vi "Read Message.vi"(4 "timeout in ms (100)":i32=100, 8 "error in (no error)":errorcluster, 11 "RemoteControl.STM in":refnum<class "RemoteControl.STM.lvclass">) -> (0 "error out":errorcluster, 1 "Message ID":u32, 2 "Message":T1, 3 "RemoteControl.STM out":refnum<class "RemoteControl.STM.lvclass">)   [LabVIEW 2016, in "RemoteControl.STM.lvclass"]
uses:
  RemoteControl.STM.lvclass
  RemoteControl/Typedefs/Message--Cluster.ctl
  <vilib>/NI/STM/TCP/TCP Read Options.ctl
  RemoteControl.STM.lvclass/RemoteControl.STM.ctl
  <vilib>/NI/STM/TCP/Read Message (TCP).vi
  <vilib>/NI/STM/NI STM.lvlib
  RemoteControl/RemoteControl.lvclass
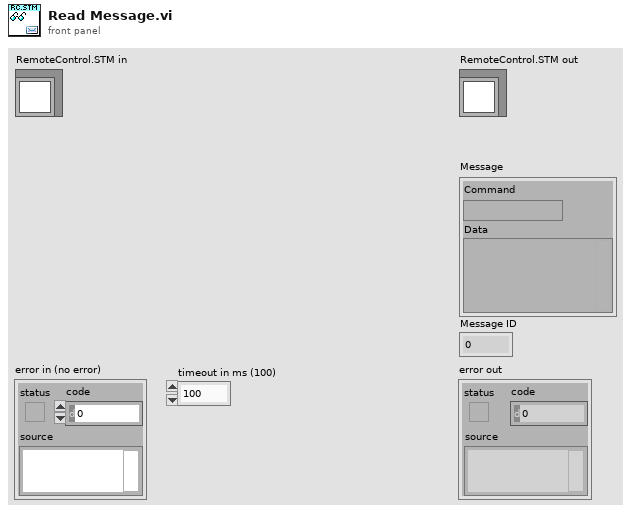
[diagram p1: front panel]
types:
  T1 = typedef "RemoteControl.lvclass/Message--Cluster.ctl" = cluster{"Command":string, "Data":variant}
  T2 = typedef "NI STM.lvlib/TCP Read Options.ctl" = cluster{"ignore timeout error":bool, "timeout ms (1000)":i32}
  T3 = typedef "NI STM.lvlib/TCP Connection Info.ctl" = cluster{"connection ID":refnum<k5>, "meta data":T4[]}
  T4 = typedef "NI STM.lvlib/MetaDataElement.ctl" = string
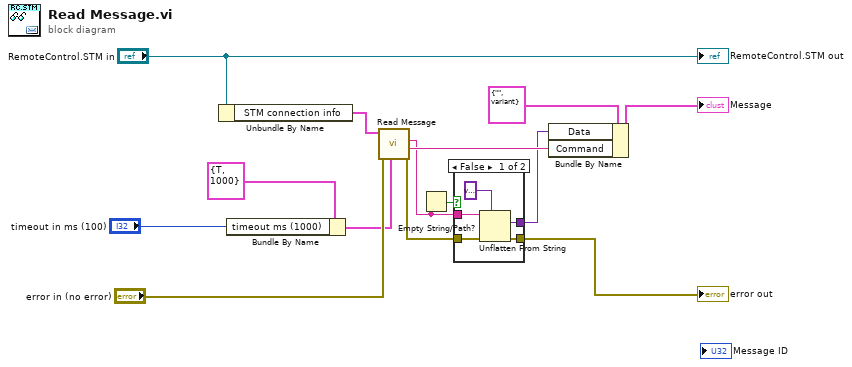
[diagram p0: block diagram]
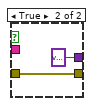
[diagram p2: hidden frame]
diagram:
  n1 = Unbundle By Name("RemoteControl.STM in") -> ("STM connection info"=w3:T3)
  n2 = Bundle By Name(cluster=T2 {"ignore timeout error"=TRUE, "timeout ms (1000)"=1000} ("options"), "timeout ms (1000)"="timeout in ms (100)") -> (w6:T2)
  n3 = call-poly <vilib>:"Read Message.vi"("options"=w6, "error in"="error in (no error)", "connection info in"=w3) -> ("error out"=w5:errorcluster, "name"=w10:T4, "data string"=w2:string)  [unwired: 3 in, 3 out]
  n4 = Empty String/Path?(string/path=w2) -> (empty?=w1:bool)
  n5 = case shown="False" w1 {
    tunnel: w5 -> [w18 w21]
    tunnel: [w17 w21] -> w13
    tunnel: [w16 variant ("Data")] -> w4
    tunnel: w2 -> [w15 _]
    frame False {
      n6 = Unflatten From String(type=variant ("Data"), binary string=w15, error in (no error)=w18) -> (value=w16:variant, error out=w17:errorcluster)  [unwired: 2 in, 1 out]
    }
    frame True {
    }
  }
  "error out" <- w13
  n7 = Bundle By Name(cluster=T1 {"Command"="", "Data"=variant} ("Message"), "Data"=w4, "Command"=w10) -> (→"Message":T1)
  "RemoteControl.STM out" <- "RemoteControl.STM in"
